vi "Update_footer.vi"(11 "Footer info":T1) -> (3 "File text out":string)   [LabVIEW 2017, in "labview-standard-library.lvlib"]
uses:
  Footer_cluster.ctl
  labview-standard-library.lvlib
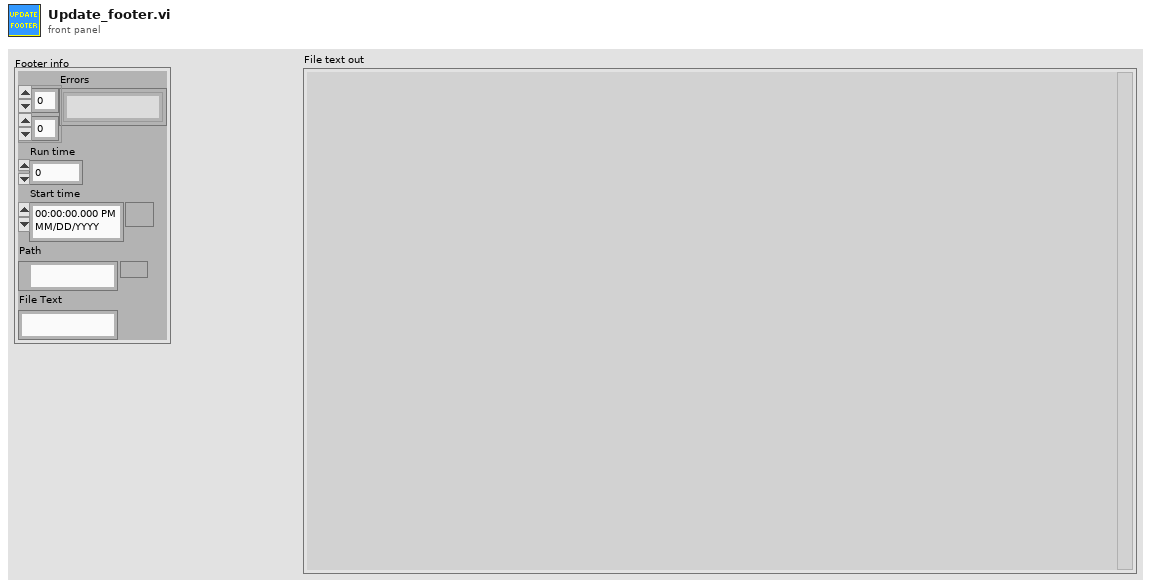
[diagram p1: front panel]
types:
  T1 = typedef "labview-standard-library.lvlib/Footer_cluster.ctl" = cluster{"Errors":string[][], "Run time":dbl, "Start time":timestamp, "Path":path, "File Text":string}
  T2 = enum16{"open", "replace", "create", "open or create", "replace or create", "replace or create with confirmation"}
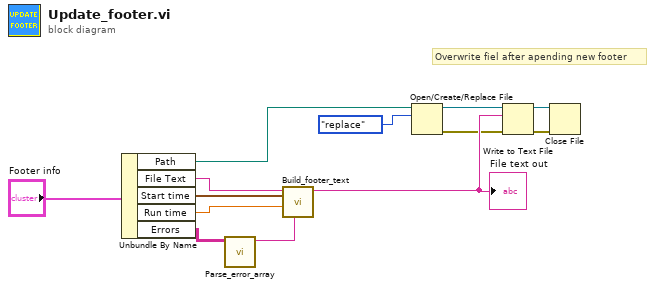
[diagram p0: block diagram]
diagram:
  # "Overwrite fiel after apending new footer"
  n1 = Unbundle By Name("Footer info") -> ("Path"=w2:path, "File Text"=w1:string, "Start time"=w11:timestamp, "Run time"=w10:dbl, "Errors"=w8:string[][])
  n2 = call "Parse_error_array.vi"("Error array"=w8) -> ("Error string"=w9:string)  [unwired: 10 in]
  n3 = call "Build_footer_text.vi"("Error string"=w9, "Run time"=w10, "Start time"=w11, "File Text"=w1) -> ("String"=w13:string)  [unwired: 7 in]
  "File text out" <- w13
  n4 = Open/Create/Replace File(file path (use dialog)=w2, operation (0:open)=T2."replace") -> (refnum out=w6:refnum<file>, error out=w7:errorcluster)  [unwired: 4 in, 1 out]
  n5 = Write to Text File(file (use dialog)=w6, text=w13, error in=w7) -> (refnum out=w3:refnum<file>, error out=w4:errorcluster)  [unwired: 1 in, 1 out]
  n6 = Close File(refnum=w3, error in=w4) -> ()  [unwired: 2 out]
